vi "Get Base Protocol.vi"(8 "error in (no error)":errorcluster, 11 "VISA in":refnum<class "VISA.lvclass">) -> (0 "error out":errorcluster, 2 "Protocol out":T1, 3 "VISA out":refnum<class "VISA.lvclass">)   [LabVIEW 2013, in "Protocol Classes.lvlib" / "VISA.lvclass"]
uses:
  VISA.lvclass
  Protocol Parent/Types/Base Protocol Type.ctl
  Protocol Parent/Protocol Parent.lvclass
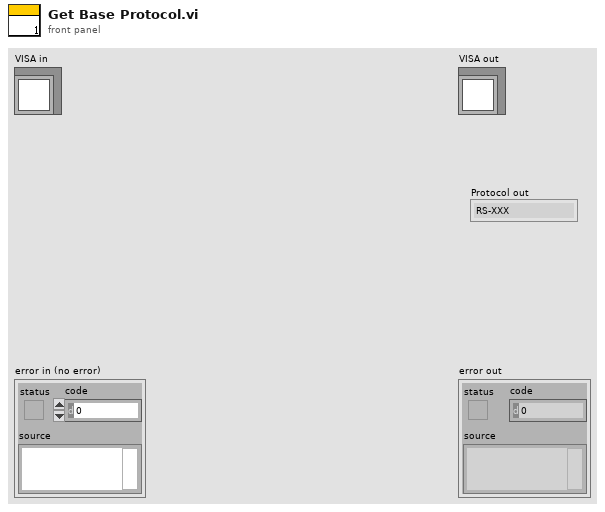
[diagram p1: front panel]
types:
  T1 = typedef "Protocol Classes.lvlib/Protocol Parent.lvclass/Base Protocol Type.ctl" = enum16{"RS-XXX", "VISA", "TCPIP", "UDP"}
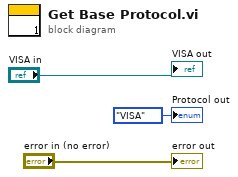
[diagram p0: block diagram]
diagram:
  "error out" <- "error in (no error)"
  "VISA out" <- "VISA in"
  "Protocol out" <- Base_Protocol_Type."VISA" ("Protocol out")
